vi "InputChannelToString.vi"(11 "Channel (1)":u16(ring)=1 items=["All Channels (0)", "1", "2", "3", "4", "5", "6", "7", "8", "9", "10", "11", "12", "13", "14", "15", "16", "A (Control Input)"]) -> (3 "Channel Str":string)   [LabVIEW 2016, in "Lake Shore 372.lvlib"]
doc: "Converts input ring text to string"
uses:
  Lake Shore 372.lvlib
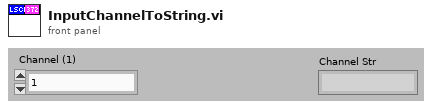
[diagram p1: front panel]
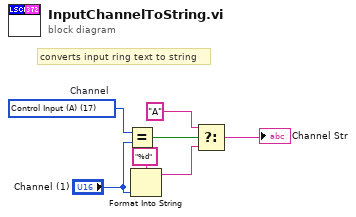
[diagram p0: block diagram]
diagram:
  w3 = u16 17 items=["All Channels", "1", "2", "3", "4", "5", "6", "7", "8", "9", "10", "11", "12", "13", "14", "15", "16", "Control Input (A)"]  # Channel
  # "converts input ring text to string"
  n1 = Equal?(x=w3, y="Channel (1)") -> (x = y?=w4:bool)
  n2 = Format Into String(format string="%d", "Channel (1)") -> (resulting string=w5:string)  [unwired: 2 in, 1 out]
  n3 = Select(t="A" ("format string"), s=w4, f=w5) -> (s? t:f=→"Channel Str":string)
